vi "SOFTMAX Vector Elements.vi"(1 "y":T1) -> (15 "softmax(y)":T1, 17 "max value":dbl, 19 "max index":i32)   [LabVIEW 2014]
uses:
  <vilib>/Analysis/Matrix/Datatypes/RealMatrix.ctl
  <vilib>/Analysis/Matrix/NI_Matrix.lvlib
panel:
  out "sum(e^y)":dbl
  out "e^y":T1
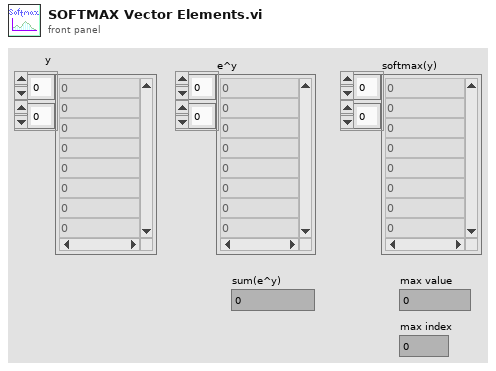
[diagram p1: front panel]
types:
  T1 = typedef "NI_Matrix.lvlib/RealMatrix.ctl" = dbl[][]
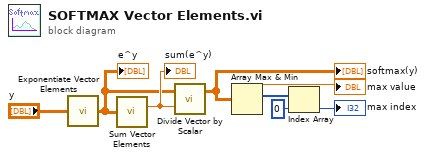
[diagram p0: block diagram]
diagram:
  n1 = call "Exponentiate Vector Elements.vi"("X"="y") -> ("exp(X)"=w4:T1)
  "e^y" <- w4
  n2 = call "Sum Vector Elements.vi"("A x B"=w4) -> ("Numeric"=w5:dbl)
  "sum(e^y)" <- w5
  n3 = call "Divide Vector by Scalar.vi"("Vector"=w4, "x"=w5) -> ("Scaled Vector"=w6:T1)  [unwired: 17 in]
  "softmax(y)" <- w6
  n4 = Array Max & Min(array=w6) -> (max value=→"max value":dbl, max index (indices)=w3:i32[])  [unwired: 2 out]
  n5 = Index Array(array=w3, index=0) -> (element=→"max index":i32)
